vi "Step_Response.vi"(6 "Times":dbl[](array[numeric]), 7 "Pressure Sets":dbl[](array[numeric]), 8 "FRP Error":errorcluster, 9 "MFCS Error":errorcluster, 10 "FRP Handle":T1, 11 "MFCS Handle":T2) -> (0 "error out":errorcluster, 1 "T":dbl[](array[numeric]), 2 "Flow Rate":dbl[](array[numeric]), 3 "Pressure Setpoint":dbl[](array[numeric]))   [LabVIEW 2016]
uses:
  <userlib>/Fluigent/Fluigent MFCS/FluigentMFCS_Full.llb/_EZmfcsRefNum.ctl
  <userlib>/Fluigent/Fluigent MFCS/FluigentMFCS_Full.llb/_EZmfcsEnum.ctl
  <userlib>/Fluigent/Fluigent FRP/FluigentFRP.llb/_frpEnum.ctl
  <userlib>/Fluigent/Fluigent MFCS/FluigentMFCS_Full.llb/MFCS_EZ Write Channel Pressure.vi
panel:
  out "Pressure set":dbl
  out "Flow Rate":dbl[](graph)
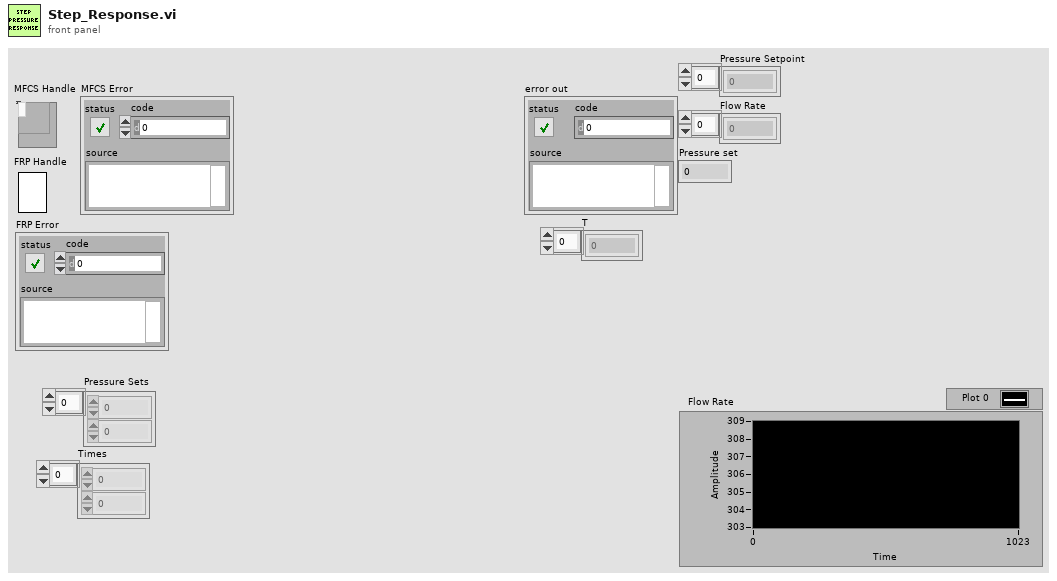
[diagram p1: front panel]
types:
  T1 = typedef "_frpRefNum" = refnum<k1>
  T2 = typedef "_EZmfcsRefNum.ctl" = refnum<k1>
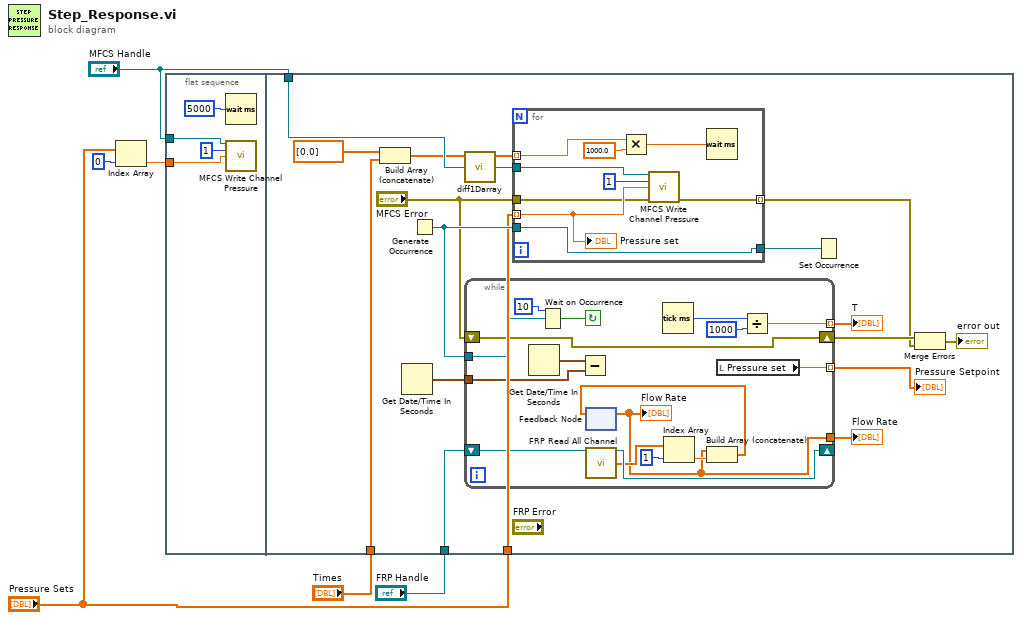
[diagram p0: block diagram]
diagram:
  n1 = Index Array(array="Pressure Sets", index=0) -> (element=w2:dbl)
  n2 = flat-sequence {
    tunnel: w2 -> [w9]
    tunnel: "MFCS Handle" -> [w8]
    tunnel: "FRP Handle" -> [w17]
    tunnel: "MFCS Handle" -> [w16]
    tunnel: "Pressure Sets" -> [w15]
    tunnel: "Times" -> [w14]
    frame #0 {
      n3 = Wait (ms)(milliseconds to wait=u32 5000) -> ()  [unwired: 1 out]
      n4 = call-poly <userlib>:"MFCS Write Channel Pressure.vi"("MFCS_EZ"=w8, "Channel Number (default=1)"=u8 1, "Pressure (mBar)"=w9) -> ()  [unwired: 11 in, 2 out]
    }
    frame #1 {
      n5 = Build Array (concatenate)(dbl[] [0.0] ("array"), w14) -> (w13:dbl[])
      n6 = Get Date/Time In Seconds() -> (seconds since 1Jan1904=w27:timestamp)
      n7 = Generate Occurrence() -> (w26:refnum<k4>)
      n8 = call "diff1Darray.vi"("Input"=w13) -> ("Diff"=w12:dbl[])  [unwired: 10 in]
      n9 = while {
        shift-right: [w37] -> w22
        shift-left: "MFCS Error" -> [w37]
        shift-right: [w51] -> _
        shift-left: w17 -> [w52]
        tunnel: w27 -> [w48]
        tunnel: [w44] -> w19
        tunnel: w26 -> [w46]
        tunnel: [w41] -> w18 mode=indexing
        tunnel: [w38] -> w11 mode=indexing
        stop <- w40 continue-if-true
        n10 = Get Date/Time In Seconds() -> (seconds since 1Jan1904=w49:timestamp)
        n11 = Wait on Occurrence(2:w46, 3:10 ("ms timeout (-1)")) -> (0:w40:bool)  [unwired: 1 in]
        n12 = Subtract(x=w49, y=w48) -> ()  [unwired: 1 out]
        n13 = feedback #1() -> (w44:dbl[])  [unwired: 1 in]
        "Flow Rate" <- w44
        n14 = call <userlib>:"FRP Read All Channel.vi"("FRP"=w52) -> ("FRP out"=w51:T1, "All Flow-Rates"=w50:dbl[])  [unwired: 12 in, 1 out]
        n15 = Tick Count (ms)() -> (millisecond timer value=w42:u32)
        n16 = Index Array(array=w50, index=1) -> (element=w47:dbl)
        n17 = Build Array (concatenate)(w44, w47) -> (w45:dbl[])
        n18 = feedback-in #1(w45) -> ()
        n19 = local read "Pressure set"() -> (w38:dbl)
        n20 = Divide(x=w42, y=u32 1000) -> (x/y=w41:dbl)
      }
      "Pressure Setpoint" <- w11
      "Flow Rate" <- w19
      "T" <- w18
      n21 = for {
        tunnel: w15 -> [w35] mode=indexing
        tunnel: w26 -> [w36]
        tunnel: [w36] -> w25
        tunnel: w16 -> [w34]
        tunnel: "MFCS Error" -> [w32]
        tunnel: [w31] -> w21 mode=indexing
        tunnel: w12 -> [w28] mode=indexing
        n22 = Multiply(x=w28, y=1000.0) -> (x*y=w30:dbl)
        n23 = call-poly <userlib>:"MFCS Write Channel Pressure.vi"("MFCS_EZ"=w34, "Channel Number (default=1)"=u8 1, "Pressure (mBar)"=w35, "error in (no error)"=w32) -> ("error out"=w31:errorcluster)  [unwired: 10 in, 1 out]
        n24 = Wait (ms)(milliseconds to wait=w30) -> ()  [unwired: 1 out]
        "Pressure set" <- w35
      }
      n25 = Set Occurrence(w25) -> ()
      n26 = Merge Errors(w22, w21) -> (→"error out":errorcluster)
    }
  }
